vi "Main.vi"() -> ()   [LabVIEW 2012]
panel:
  in  "Stop Button":bool
  out "3D Picture":refnum<vi>(3d-picture)
  in  "Horizontal Pointer Slide 6":dbl(slide)=30.0 min=30.0 max=40.0 scale=30.0..40.0
  in  "Horizontal Pointer Slide 5":dbl(slide)=30.0 min=30.0 max=40.0 scale=30.0..40.0
  in  "Horizontal Pointer Slide 4":dbl(slide)=30.0 min=30.0 max=40.0 scale=30.0..40.0
  in  "Horizontal Pointer Slide 3":dbl(slide)=30.0 min=30.0 max=40.0 scale=30.0..40.0
  in  "Horizontal Pointer Slide 2":dbl(slide) scale=30.0..40.0
  in  "Horizontal Pointer Slide":dbl(slide) scale=30.0..40.0
  # "3D Sensor Mapping"
  # "Sensors"
  # "3D View"
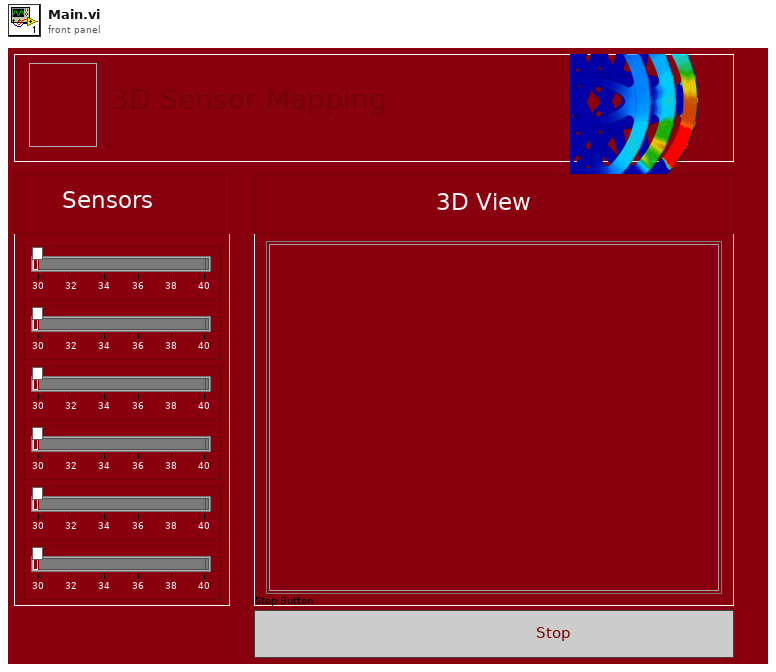
[diagram p1: front panel]
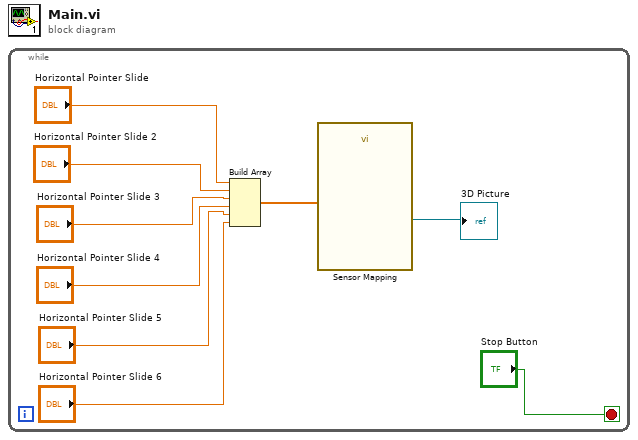
[diagram p0: block diagram]
diagram:
  n1 = while {
    stop <- "Stop Button" stop-if-true
    n2 = Build Array("Horizontal Pointer Slide", "Horizontal Pointer Slide 2", "Horizontal Pointer Slide 3", "Horizontal Pointer Slide 4", "Horizontal Pointer Slide 5", "Horizontal Pointer Slide 6") -> (w3:dbl[])
    n3 = call "Sensor Mapping"("Sensor Values"=w3) -> ("Scene Ref Out"=→"3D Picture":refnum<vi>)  [unwired: 9 in, 1 out]
  }
